vi "Send Subscribe Message.vi"(8 "error in":errorcluster, 10 "Topic":string, 11 "Actor Class":T1) -> (0 "error out":errorcluster)   [LabVIEW 2013]
uses:
  Actor Private Data.ctl
  <vilib>/LabVIEW Open Source Project/MQTT Client/Client class/Client.lvclass
  Actor Private Events -- cluster.ctl
  Payload -- cluster.ctl
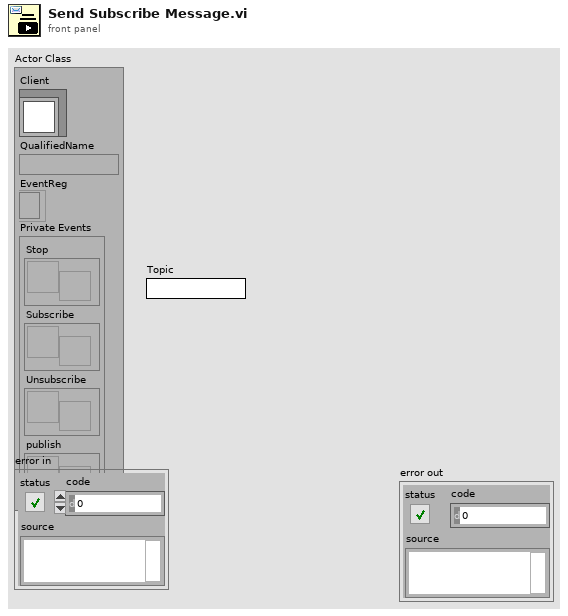
[diagram p1: front panel]
types:
  T1 = typedef "Actor Private Data.ctl" = cluster{"Client":refnum<class "Client.lvclass">, "QualifiedName":string, "EventReg":refnum<event-registration>, "Private Events":T2}
  T2 = typedef "Actor Private Events -- cluster.ctl" = cluster{"Stop":refnum<user-event>, "Subscribe":refnum<user-event>, "Unsubscribe":refnum<user-event>, "publish":refnum<user-event>}
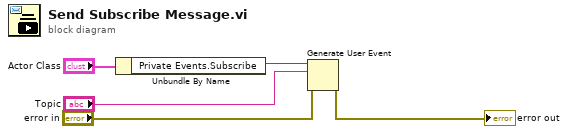
[diagram p0: block diagram]
diagram:
  n1 = Unbundle By Name("Actor Class") -> ("Private Events.Subscribe"=w4:refnum<user-event>)
  n2 = Generate User Event(user event=w4, event data cluster="Topic", error in="error in") -> (error out=→"error out":errorcluster)  [unwired: 1 in, 1 out]
